vi "Set Help Control Position.vi"(8 "error in (no error)":errorcluster, 10 "Width":u32, 11 "String in":refnum<vi>) -> (0 "error out":errorcluster, 3 "String out":refnum<vi>)   [LabVIEW 2018]
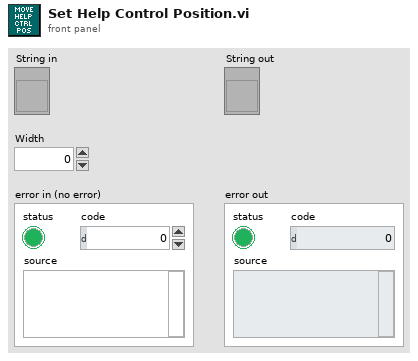
[diagram p1: front panel]
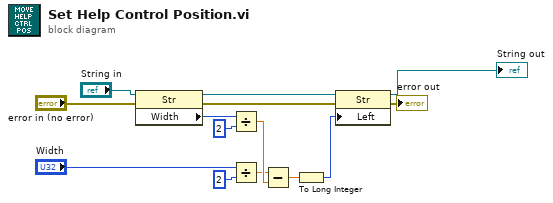
[diagram p0: block diagram]
diagram:
  n1 = property class="Str"(reference="String in", error in="error in (no error)") -> (reference out=w3:refnum<vi>, error out=w4:errorcluster, "Width"=w6:u32)
  n2 = Divide(x=w6, y=u32 2) -> (x/y=w14:dbl)
  n3 = Divide(x="Width", y=u32 2) -> (x/y=w9:dbl)
  n4 = Subtract(x=w9, y=w14) -> (x-y=w10:dbl)
  n5 = To Long Integer(number=w10) -> (32bit integer=w13:i32)
  n6 = property class="Str"(reference=w3, error in=w4, "Left"=w13) -> (reference out=→"String out":refnum<vi>, error out=→"error out":errorcluster)
